vi "CRYReport Pic Insert Text.vi"(9 "sData":string, 11 "TXTextControl":refnum<k7>) -> ()   [LabVIEW 2013]
uses:
  CRYReport Global.vi
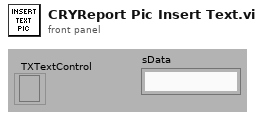
[diagram p1: front panel]
types:
  T1 = enum16{"open", "open or create", "create or replace", "create", "open (read only)"}
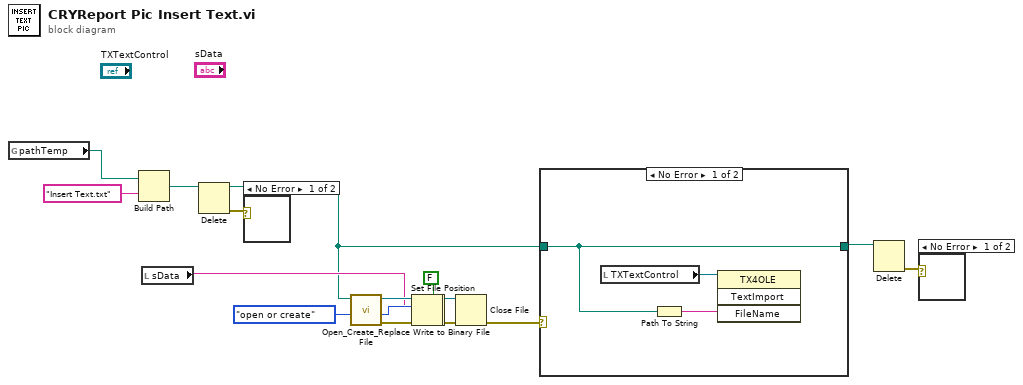
[diagram p0: block diagram]
diagram:
  n1 = global read "CRYReport Global.vi" "pathTemp"() -> (w8:path)
  n2 = Build Path(base path=w8, name or relative path="Insert Text.txt" ("name")) -> (appended path=w5:path)
  n3 = local read "sData"() -> (w7:string)
  n4 = Delete(path (use dialog)=w5) -> (deleted path=w4:path, error out=w3:errorcluster)  [unwired: 4 in, 1 out]
  n5 = case shown="No Error" w3 {
    frame No Error {
    }
    frame Error {
    }
  }
  n6 = call <vilib>:"Open_Create_Replace File.vi"("function (open:0)"=T1."open or create", "file path"=w4) -> ("error out"=w16:errorcluster, "file size (bytes)"=w14:i32, "refnum"=w15:refnum<file>)  [unwired: 6 in, 1 out]
  n7 = Set File Position(offset (in bytes) (0)=w14, refnum=w15, error in=w16) -> (refnum out=w11:refnum<file>, error out=w10:errorcluster)  [unwired: 1 in]
  n8 = Write to Binary File(file (use dialog)=w11, data=w7, error in=w10, 5:FALSE ("prepend array or string size? (T)")) -> (refnum out=w12:refnum<file>, error out=w13:errorcluster)  [unwired: 2 in, 1 out]
  n9 = Close File(refnum=w12, error in=w13) -> (error out=w6:errorcluster)  [unwired: 1 out]
  n10 = case shown="No Error" w6 {
    tunnel: w4 -> [w19 w22]
    tunnel: [w19 w22] -> w1
    frame No Error {
      n11 = local read "TXTextControl"() -> (w21:refnum<k7>)
      n12 = Path To String(path=w19) -> (string=w20:string)
      n13 = invoke class="TX4OLE" method="TextImport"(reference=w21, "FileName"=w20) -> ()  [unwired: 2 in, 4 out]
    }
    frame Error {
    }
  }
  n14 = Delete(path (use dialog)=w1) -> (error out=w2:errorcluster)  [unwired: 4 in, 2 out]
  n15 = case shown="No Error" w2 {
    frame No Error {
    }
    frame Error {
    }
  }
